vi "one_stop_button.vi"() -> ()   [LabVIEW 2019]
panel:
  in  "stop":bool
  out "Numeric 4":i32
  out "Numeric 3":i32
  out "Numeric 2":i32
  out "Numeric":i32
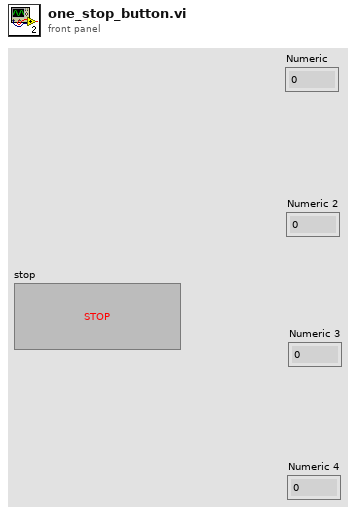
[diagram p1: front panel]
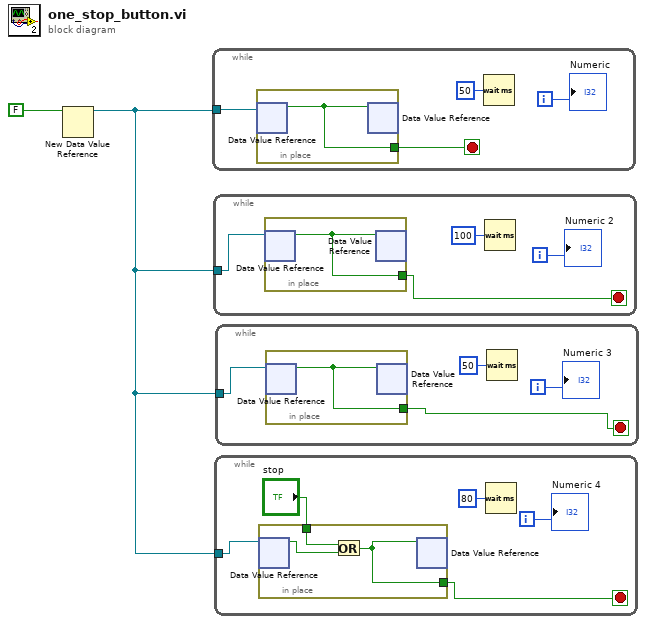
[diagram p0: block diagram]
diagram:
  n1 = New Data Value Reference(data value=FALSE) -> (data value reference=w1:refnum<data-value>)  [unwired: 1 in, 1 out]
  n2 = while {
    tunnel: w1 -> [w4]
    i -> [w6]
    stop <- w3 stop-if-true
    n3 = in-place {
      in-place-border: [w7] -> w3
      n4 = in-place-dvr #1(w4) -> (w7:bool)  [unwired: 1 out]
      n5 = in-place-dvr #1(w7) -> ()  [unwired: 2 out]
    }
    n6 = Wait (ms)(milliseconds to wait=u32 50) -> ()  [unwired: 1 out]
    "Numeric" <- w6
  }
  n7 = while {
    tunnel: w1 -> [w9]
    i -> [w11]
    stop <- w8 stop-if-true
    n8 = in-place {
      in-place-border: [w12] -> w8
      n9 = in-place-dvr #2(w9) -> (w12:bool)  [unwired: 1 out]
      n10 = in-place-dvr #2(w12) -> ()  [unwired: 2 out]
    }
    n11 = Wait (ms)(milliseconds to wait=u32 100) -> ()  [unwired: 1 out]
    "Numeric 2" <- w11
  }
  n12 = while {
    tunnel: w1 -> [w15]
    i -> [w17]
    stop <- w13 stop-if-true
    n13 = in-place {
      in-place-border: [w18] -> w13
      in-place-border: "stop" -> [w19]
      n14 = in-place-dvr #3(w15) -> (w20:bool)  [unwired: 1 out]
      n15 = Or(x=w19, y=w20) -> (x .or. y?=w18:bool)
      n16 = in-place-dvr #3(w18) -> ()  [unwired: 2 out]
    }
    n17 = Wait (ms)(milliseconds to wait=u32 80) -> ()  [unwired: 1 out]
    "Numeric 4" <- w17
  }
  n18 = while {
    tunnel: w1 -> [w22]
    i -> [w24]
    stop <- w21 stop-if-true
    n19 = in-place {
      in-place-border: [w25] -> w21
      n20 = in-place-dvr #4(w22) -> (w25:bool)  [unwired: 1 out]
      n21 = in-place-dvr #4(w25) -> ()  [unwired: 2 out]
    }
    n22 = Wait (ms)(milliseconds to wait=u32 50) -> ()  [unwired: 1 out]
    "Numeric 3" <- w24
  }
